vi "Run Continuous Analog.vi"(9 "Initialize first run":bool=TRUE, 10 "Samples / channel":i32=8192, 11 "ADALM2000 Handler":u64 caption="Instrument Handle Out") -> (0 "Waveform 2":waveform(dbl), 1 "Waveform":waveform(dbl), 3 "ADALM2000 Handler 2":u64 caption="Instrument Handle Out")   [LabVIEW 2022 SP3]
uses:
  <vilib>/Waveform/WDTOps.llb/WDT Append Waveforms DBL.vi
  libm2k_lv.dll
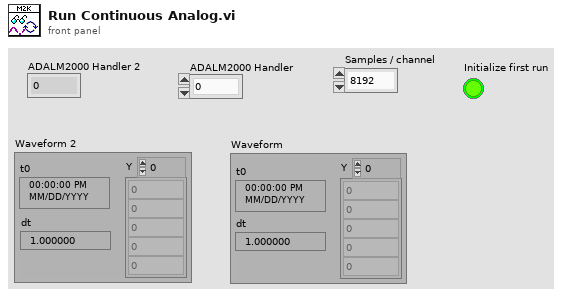
[diagram p1: front panel]
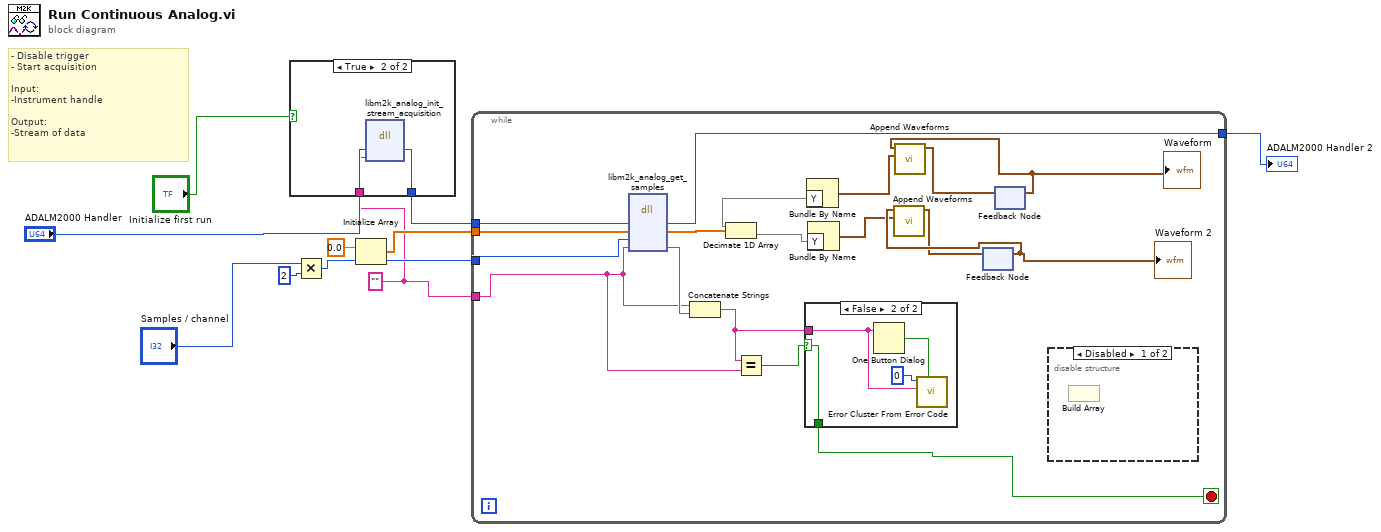
[diagram p0: block diagram]
diagram:
  w3 = ""
  # "- Disable trigger\n- Start acquisition\n\nInput:\n-Instrument handle\n\nOutput:\n-Stream of data"
  n1 = case shown="True" "Initialize first run" {
    tunnel: "ADALM2000 Handler" -> [w11 w14]
    tunnel: [w11 w13] -> w4
    tunnel: w3 -> [_ w12]
    frame False {
    }
    frame True {
      n2 = dll-call lib="libm2k_lv.*" fn="libm2k_analog_init_stream_acquisition"("instance"=w14, "err"=w12) -> ("instance"=w13:u64)  [unwired: 5 in, 2 out]
    }
  }
  n3 = Multiply(x="Samples / channel", y=2) -> (x*y=w7:i32)
  n4 = Initialize Array(0.0, w7) -> (w8:dbl[])
  n5 = while {
    tunnel: w4 -> [w32]
    tunnel: w8 -> [w31]
    tunnel: w7 -> [w30]
    tunnel: w3 -> [w26]
    tunnel: [w15] -> w2
    stop <- w19 stop-if-true
    n6 = dll-call lib="libm2k_lv.*" fn="libm2k_analog_get_samples"("instance"=w32, "analog_samples"=w31, "nb_samples"=w30, "err"=w26) -> ("instance"=w15:u64, "analog_samples"=w28:dbl[], "err"=w29:string)  [unwired: 5 in, 2 out]
    n7 = Concatenate Strings(w26, w29) -> (w25:string)
    n8 = Decimate 1D Array(w28) -> (w21:dbl[], w20:dbl[])
    n9 = Equal?(x=w25, y=w26) -> (x = y?=w27:bool)
    n10 = case shown="False" w27 {
      selector: w27 -> [w33 w34]
      tunnel: w25 -> [_ w36]
      tunnel: [w33 w34] -> w19
      frame True {
      }
      frame False {
        n11 = One Button Dialog(message=w36) -> (true=w35:bool)  [unwired: 1 in]
        n12 = call <vilib>:"Error Cluster From Error Code.vi"("show call chain? (False)"=w35, "error message (\"\")"=w36, "error code (0)"=0) -> ()  [unwired: 6 in, 1 out]
      }
    }
    n13 = Bundle By Name("Y"=w21) -> (w24:waveform(dbl))  [unwired: 1 in]
    n14 = Bundle By Name("Y"=w20) -> (w16:waveform(dbl))  [unwired: 1 in]
    n15 = feedback #1() -> (w18:waveform(dbl))  [unwired: 1 in]
    "Waveform 2" <- w18
    n16 = call-poly <vilib>:"Append Waveforms.vi"("waveform B"=w16, "waveform A"=w18) -> ("waveform out"=w17:waveform(dbl))  [unwired: 8 in, 1 out]
    n17 = feedback-in #1(w17) -> ()
    n18 = feedback #2() -> (w22:waveform(dbl))  [unwired: 1 in]
    "Waveform" <- w22
    n19 = call-poly <vilib>:"Append Waveforms.vi"("waveform B"=w24, "waveform A"=w22) -> ("waveform out"=w23:waveform(dbl))  [unwired: 8 in, 1 out]
    n20 = feedback-in #2(w23) -> ()
    n21 = disable-structure shown="Disabled" {
      frame Disabled {
        n22 = Build Array() -> ()  [unwired: 2 in, 1 out]
      }
      frame Enabled {
      }
    }
  }
  "ADALM2000 Handler 2" <- w2
